vi "Transpose 3D(boolean).vi"(8 "error in (no error)":errorcluster, 10 "Transpose":T1(ring), 11 "Input Array":bool[][][](array[boolean])) -> (0 "error out":errorcluster, 3 "Output Array":bool[][][](array[boolean]))   [LabVIEW 2018]
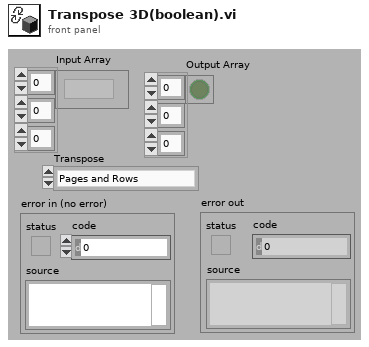
[diagram p1: front panel]
types:
  T1 = enum16{"Pages and Rows", "Pages and Columns", "Rows and Columns"}
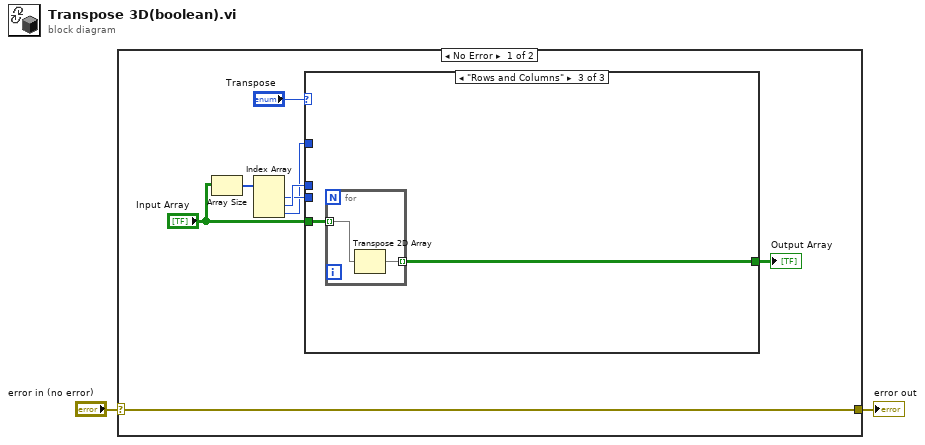
[diagram p0: block diagram]
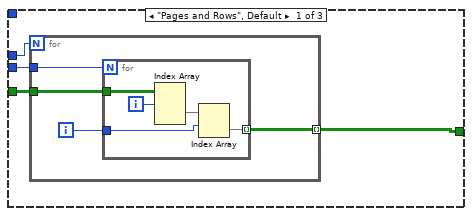
[diagram p2: hidden frame]
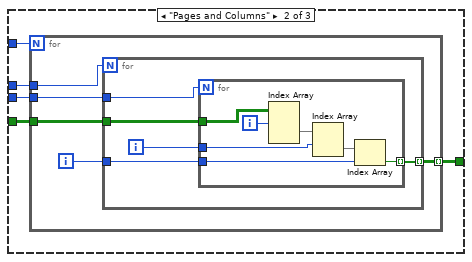
[diagram p3: hidden frame]
diagram:
  n1 = case shown="No Error" "error in (no error)" {
    selector: "error in (no error)" -> [w5 w50]
    tunnel: [w5 w50] -> w1
    frame No Error {
      n2 = Array Size(array="Input Array") -> (size(s)=w10:i32[])
      n3 = Index Array(array=w10) -> (element #1=w8:i32, element #2=w9:i32, element #3=w6:i32)  [unwired: 3 in]
      n4 = case shown="\"Rows and Columns\"" "Transpose" {
        tunnel: "Input Array" -> [w14 w28 w47]
        tunnel: w9 -> [w13 w24 _]
        tunnel: w8 -> [w12 w26 _]
        tunnel: [w11 w27 w46] -> w3
        tunnel: w6 -> [_ w25 _]
        frame "Pages and Rows", Default {
          n5 = for {
            N: w13 -> [_]
            tunnel: w14 -> [w18]
            tunnel: w12 -> [w17]
            tunnel: [w15] -> w11 mode=indexing
            i -> [w16]
            n6 = for {
              N: w17 -> [_]
              tunnel: w18 -> [w23]
              tunnel: w16 -> [w20]
              tunnel: [w19] -> w15 mode=indexing
              i -> [w22]
              n7 = Index Array(array=w23, index (dim 0)=w22) -> (element=w21:bool[][])  [unwired: 2 in]
              n8 = Index Array(array=w21, index (row)=w20) -> (element=w19:bool[])  [unwired: 1 in]
            }
          }
        }
        frame "Pages and Columns" {
          n9 = for {
            N: w25 -> [_]
            tunnel: w28 -> [w33]
            tunnel: [w31] -> w27 mode=indexing
            tunnel: w26 -> [w30]
            tunnel: w24 -> [w29]
            i -> [w32]
            n10 = for {
              N: w29 -> [_]
              tunnel: w33 -> [w38]
              tunnel: w32 -> [w36]
              tunnel: [w35] -> w31 mode=indexing
              tunnel: w30 -> [w34]
              i -> [w37]
              n11 = for {
                N: w34 -> [_]
                tunnel: w38 -> [w45]
                tunnel: w37 -> [w40]
                tunnel: w36 -> [w39]
                tunnel: [w42] -> w35 mode=indexing
                i -> [w41]
                n12 = Index Array(array=w45, index (dim 0)=w41) -> (element=w44:bool[][])  [unwired: 2 in]
                n13 = Index Array(array=w44, index (row)=w40) -> (element=w43:bool[])  [unwired: 1 in]
                n14 = Index Array(array=w43, index=w39) -> (element=w42:bool)
              }
            }
          }
        }
        frame "Rows and Columns" {
          n15 = for {
            tunnel: w47 -> [w49] mode=indexing
            tunnel: [w48] -> w46 mode=indexing
            n16 = Transpose 2D Array(2D array=w49) -> (transposed array=w48:bool[][])
          }
        }
      }
      "Output Array" <- w3
    }
    frame Error {
    }
  }
  "error out" <- w1
